vi "simx Get Vision Sensor Depth Buffer.vi"(6 "operationMode":i32, 7 "buffer":sgl, 8 "error in (no error)":errorcluster, 9 "resolution":i32, 10 "sensorHandle":i32, 11 "clientID":i32) -> (0 "error out":errorcluster, 1 "resolution out":i32, 3 "function return":i32, 5 "buffer out":sgl)   [LabVIEW 2019, in "PXL_V-REP.lvlib"]
doc: "EXTAPI_DLLEXPORT simxInt simxGetVisionSensorDepthBuffer(simxInt clientID,simxInt sensorHandle,simxInt* resolution,simxFloat** buffer,simxInt operationMode);"
uses:
  PXL_V-REP.lvlib
  <userlib>/V-REP/remoteApi.dll
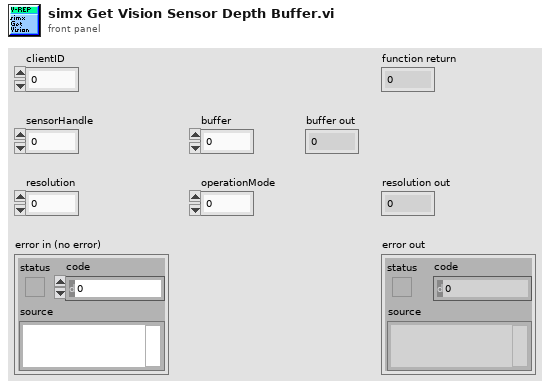
[diagram p1: front panel]
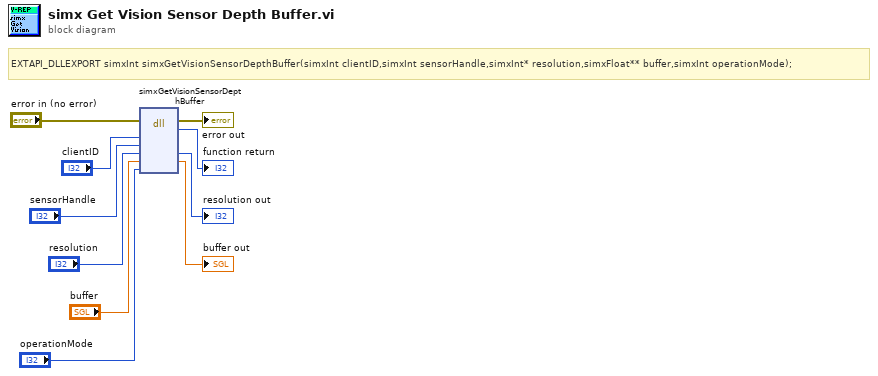
[diagram p0: block diagram]
diagram:
  # "EXTAPI_DLLEXPORT simxInt simxGetVisionSensorDepthBuffer(simxInt clientID,simxInt sensorHandle,simxInt* resolution,simxFloat** buffer,simxInt operationMode);"
  n1 = dll-call lib="C:/Program Files (x86)/National Instruments/LabVIEW 2019/user.lib/V-REP/remoteApi.*" fn="simxGetVisionSensorDepthBuffer"(error in="error in (no error)", "clientID"="clientID", "sensorHandle"="sensorHandle", "resolution"="resolution", "buffer"="buffer", "operationMode"="operationMode") -> (error out=→"error out":errorcluster, →"function return":i32, "resolution"=→"resolution out":i32, "buffer"=→"buffer out":sgl)  [unwired: 5 in, 1 out]
